vi "Set Light RGB By ID.vi"(7 "ID":u8, 8 "Error In":errorcluster, 10 "Color":u32(colorbox), 11 "Hue Config":T1) -> (0 "Error Out":errorcluster, 3 "Hue Config":T1)   [LabVIEW 2013, in "LVH-Hue.lvlib"]
uses:
  LVH-Hue.lvlib
  Type Defs/Hue Ref.ctl
  <vilib>/httpClient/ClientHandle.ctl
  Type Defs/Light.ctl
  <vilib>/httpClient/LabVIEWHTTPClient.lvlib
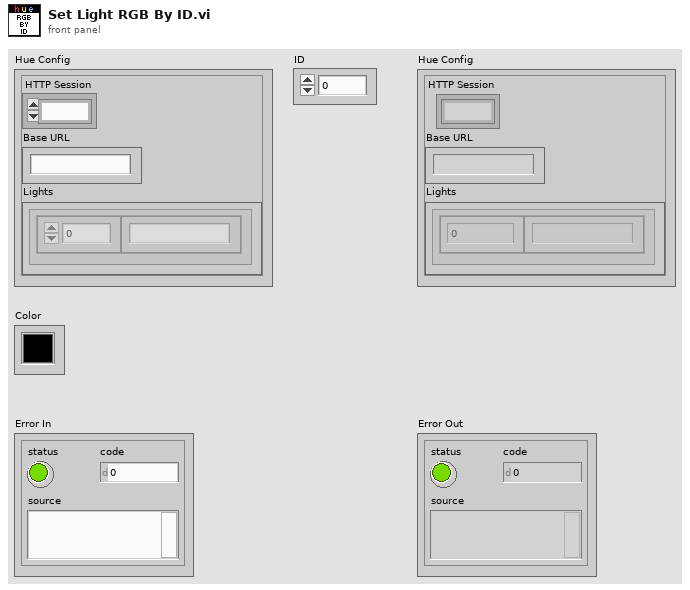
[diagram p1: front panel]
types:
  T1 = typedef "LVH-Hue.lvlib/Hue Ref.ctl" = cluster{"HTTP Session":T2, "Base URL":string, "Lights":T3[]}
  T2 = typedef "LabVIEWHTTPClient.lvlib/ClientHandle.ctl" = refnum<k1>
  T3 = typedef "LVH-Hue.lvlib/Light.ctl" = cluster{"ID":i32, "Name":string}
  T4 = typedef "LVH-Hue.lvlib/HSB.ctl" = cluster{"Hue":u16, "Saturation":u8, "Brightness":u8}
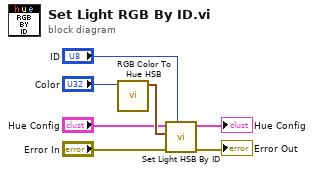
[diagram p0: block diagram]
diagram:
  n1 = call "RGB Color To Hue HSB.vi"("Color"="Color") -> ("HSB"=w7:T4)  [unwired: 10 in]
  n2 = call "Set Light HSB By ID.vi"("ID"="ID", "Error In"="Error In", "HSB"=w7, "Hue Config"="Hue Config") -> ("Error Out"=→"Error Out":errorcluster, "Hue Config"=→"Hue Config":T1)  [unwired: 6 in]
